vi "2024_day05.vi"() -> ()   [LabVIEW 2023]
uses:
  <userlib>/_OpenG.lib/array/array.llb/Search 1D Array (I32)__ogtk.vi
  <userlib>/_OpenG.lib/string/string.llb/openg_string.lvlib
  <userlib>/_OpenG.lib/array/array.llb/openg_array.lvlib
panel:
  out "Result - Task 2":i32
  out "Result - Task 1":i32
  in  "Switch":bool caption="Ex. Data  vs.  User Data"
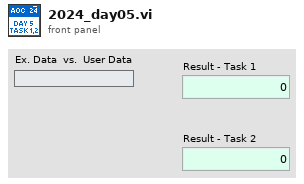
[diagram p1: front panel]
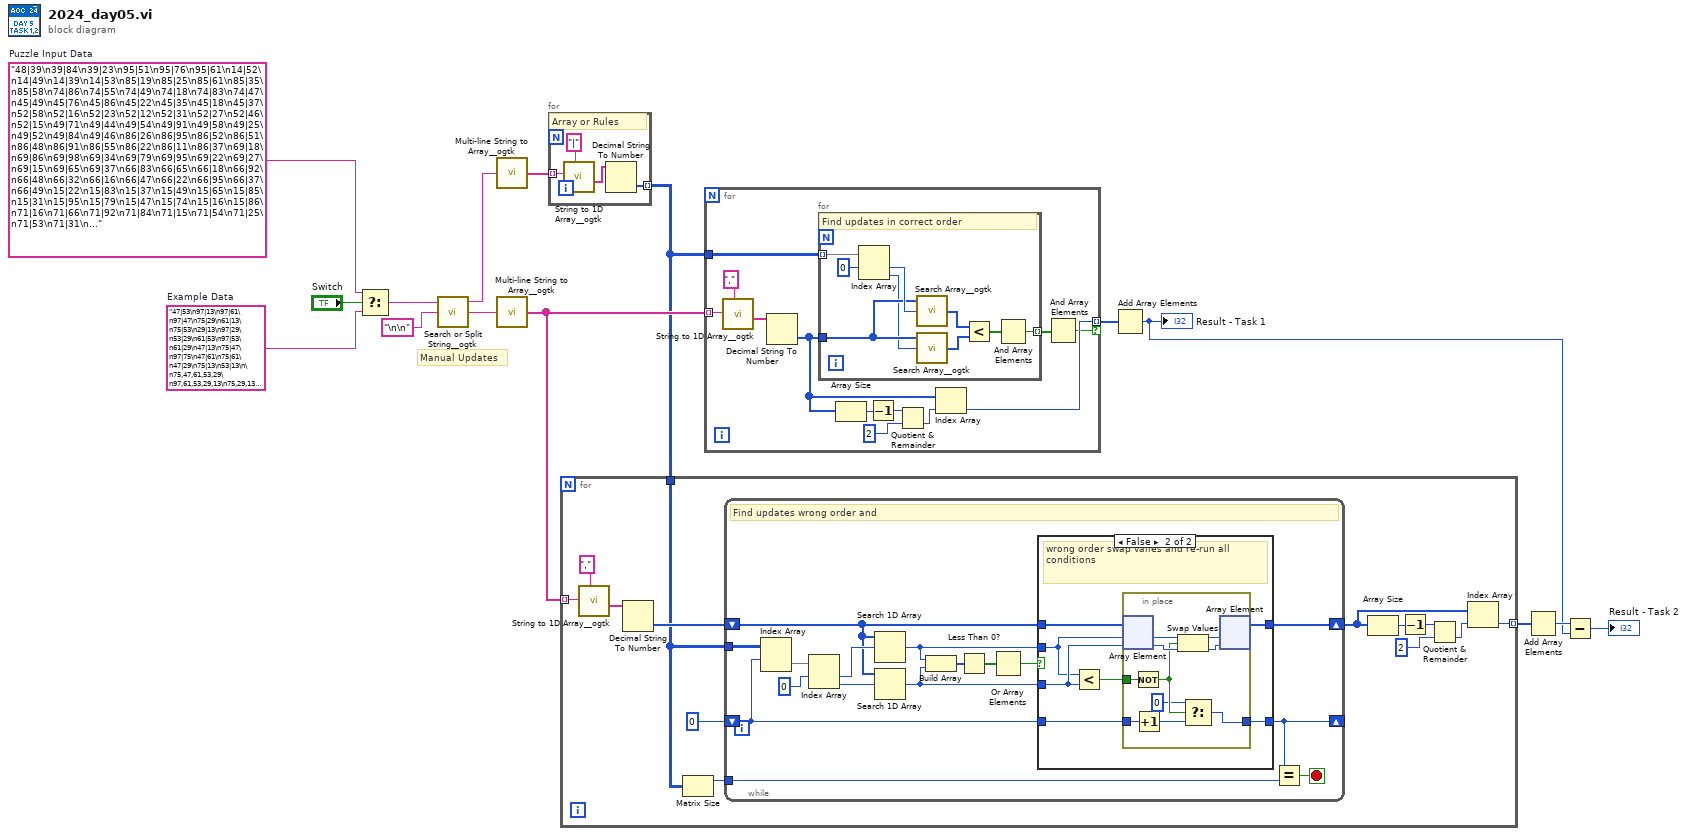
[diagram p0: block diagram]
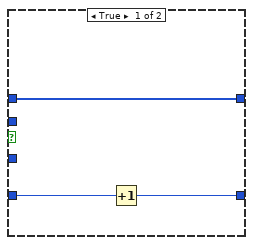
[diagram p2: hidden frame]
diagram:
  w13 = "48|39\n39|84\n39|23\n95|51\n95|76\n95|61\n14|52\n14|49\n14|39\n14|53\n85|19\n85|25\n85|61\n85|35\n85|58\n74|86\n74|55\n74|49\n74|18\n74|83\n74|47\n45|49\n45|76\n45|86\n45|22\n45|35\n45|18\n45|37\n52|58\n52|16\n52|23\n52|12\n52|31\n52|27\n52|46\n52|15\n49|71\n49|44\n49|54\n49|91\n49|58\n49|25\n49|52\n49|84\n49|46\n86|26\n86|95\n86|52\n86|51\n86|48\n86|91\n86|55\n86|22\n86|11\n86|37\n69|18\n69|86\n69|98\n69|34\n69|79\n69|95\n69|22\n69|27\n69|15\n69|65\n69|37\n66|83\n66|65\n66|18\n66|92\n66|48\n66|32\n66|16\n66|47\n66|22\n66|95\n66|37\n66|49\n15|22\n15|83\n15|37\n15|49\n15|65\n15|85\n15|31\n15|95\n15|79\n15|47\n15|74\n15|16\n15|86\n71|16\n71|66\n71|92\n71|84\n71|15\n71|54\n71|25\n71|53\n71|31\n71|98\n71|46\n71|69\n71|74\n71|58\n79|49\n79|34\n79|86\n79|26\n79|18\n79|14\n79|22\n79|91\n79|77\n79|48\n79|37\n79|52\n79|95\n79|35\n79|74\n76|39\n76|84\n76|94\n76|77\n76|12\n76|24\n76|46\n76|69\n76|15\n76|53\n76|23\n76|19\n76|52\n76|11\n76|66\n76|25\n19|94\n19|79\n19|71\n19|92\n19|66\n19|16\n19|53\n19|45\n19|69\n19|31\n19|24\n19|25\n19|12\n19|54\n19|84\n19|58\n19|98\n11|25\n11|27\n11|84\n11|12\n11|24\n11|66\n11|19\n11|51\n11|69\n11|16\n11|53\n11|94\n11|58\n11|44\n11|23\n11|39\n11|35\n11|52\n92|37\n92|91\n92|31\n92|48\n92|76\n92|14\n92|34\n92|55\n92|32\n92|85\n92|86\n92|98\n92|83\n92|49\n92|18\n92|26\n92|95\n92|11\n92|74\n23|16\n23|18\n23|86\n23|74\n23|92\n23|66\n23|79\n23|55\n23|45\n23|47\n23|26\n23|37\n23|15\n23|24\n23|12\n23|98\n23|34\n23|48\n23|65\n23|27\n37|51\n37|61\n37|26\n37|47\n37|49\n37|84\n37|52\n37|34\n37|55\n37|39\n37|14\n37|19\n37|77\n37|35\n37|58\n37|91\n37|83\n37|76\n37|85\n37|11\n37|32\n55|44\n55|19\n55|52\n55|39\n55|84\n55|54\n55|32\n55|47\n55|71\n55|51\n55|83\n55|35\n55|91\n55|85\n55|76\n55|11\n55|58\n55|61\n55|53\n55|49\n55|25\n55|77\n27|48\n27|18\n27|65\n27|34\n27|74\n27|37\n27|47\n27|98\n27|55\n27|83\n27|79\n27|16\n27|86\n27|85\n27|45\n27|66\n27|22\n27|49\n27|15\n27|26\n27|14\n27|92\n27|95\n51|16\n51|84\n51|54\n51|77\n51|27\n51|94\n51|66\n51|23\n51|19\n51|25\n51|71\n51|65\n51|15\n51|52\n51|39\n51|44\n51|46\n51|24\n51|12\n51|31\n51|92\n51|69\n51|58\n51|53\n83|32\n83|52\n83|35\n83|76\n83|94\n83|44\n83|84\n83|14\n83|71\n83|77\n83|61\n83|12\n83|85\n83|23\n83|39\n83|51\n83|19\n83|54\n83|25\n83|49\n83|11\n83|53\n83|58\n83|91\n94|66\n94|15\n94|74\n94|12\n94|55\n94|86\n94|16\n94|69\n94|26\n94|45\n94|34\n94|65\n94|98\n94|18\n94|23\n94|48\n94|46\n94|92\n94|37\n94|31\n94|22\n94|27\n94|24\n94|79\n54|15\n54|26\n54|92\n54|46\n54|69\n54|22\n54|23\n54|66\n54|24\n54|74\n54|31\n54|37\n54|16\n54|48\n54|34\n54|94\n54|65\n54|79\n54|45\n54|18\n54|12\n54|27\n54|86\n54|98\n58|23\n58|31\n58|48\n58|25\n58|79\n58|65\n58|15\n58|24\n58|16\n58|54\n58|86\n58|22\n58|94\n58|46\n58|27\n58|12\n58|45\n58|69\n58|92\n58|74\n58|66\n58|44\n58|98\n58|18\n61|65\n61|46\n61|54\n61|19\n61|77\n61|52\n61|39\n61|25\n61|66\n61|12\n61|24\n61|94\n61|44\n61|51\n61|27\n61|15\n61|69\n61|71\n61|23\n61|84\n61|58\n61|92\n61|16\n61|53\n77|53\n77|84\n77|24\n77|58\n77|65\n77|12\n77|31\n77|92\n77|46\n77|23\n77|66\n77|27\n77|25\n77|39\n77|19\n77|71\n77|16\n77|45\n77|52\n77|94\n77|69\n77|44\n77|54\n77|15\n32|35\n32|61\n32|51\n32|71\n32|91\n32|53\n32|46\n32|39\n32|52\n32|11\n32|23\n32|77\n32|76\n32|12\n32|27\n32|54\n32|94\n32|19\n32|58\n32|44\n32|25\n32|24\n32|69\n32|84\n31|85\n31|79\n31|35\n31|91\n31|86\n31|18\n31|76\n31|98\n31|55\n31|45\n31|95\n31|11\n31|49\n31|22\n31|14\n31|74\n31|34\n31|32\n31|26\n31|48\n31|83\n31|61\n31|37\n31|47\n34|26\n34|77\n34|85\n34|47\n34|61\n34|52\n34|19\n34|11\n34|58\n34|91\n34|35\n34|95\n34|39\n34|25\n34|14\n34|53\n34|71\n34|84\n34|76\n34|51\n34|83\n34|55\n34|49\n34|32\n46|22\n46|26\n46|98\n46|27\n46|45\n46|15\n46|83\n46|86\n46|24\n46|18\n46|65\n46|79\n46|34\n46|16\n46|55\n46|74\n46|95\n46|66\n46|92\n46|37\n46|47\n46|48\n46|69\n46|31\n26|53\n26|95\n26|35\n26|47\n26|19\n26|76\n26|83\n26|55\n26|11\n26|51\n26|77\n26|52\n26|39\n26|71\n26|91\n26|44\n26|32\n26|84\n26|85\n26|14\n26|49\n26|61\n26|25\n26|58\n91|24\n91|23\n91|94\n91|69\n91|46\n91|27\n91|76\n91|58\n91|53\n91|11\n91|19\n91|39\n91|52\n91|61\n91|84\n91|51\n91|25\n91|54\n91|77\n91|35\n91|44\n91|12\n91|15\n91|71\n53|48\n53|69\n53|44\n53|94\n53|92\n53|66\n53|79\n53|98\n53|31\n53|27\n53|45\n53|15\n53|16\n53|22\n53|12\n53|86\n53|54\n53|24\n53|58\n53|23\n53|74\n53|46\n53|65\n53|25\n12|74\n12|16\n12|65\n12|66\n12|95\n12|31\n12|34\n12|37\n12|47\n12|24\n12|98\n12|92\n12|15\n12|22\n12|69\n12|86\n12|27\n12|46\n12|55\n12|26\n12|45\n12|18\n12|79\n12|48\n24|34\n24|15\n24|26\n24|27\n24|95\n24|55\n24|37\n24|14\n24|74\n24|48\n24|31\n24|66\n24|45\n24|98\n24|18\n24|86\n24|92\n24|16\n24|65\n24|47\n24|83\n24|79\n24|22\n24|85\n84|54\n84|98\n84|53\n84|46\n84|58\n84|23\n84|22\n84|12\n84|16\n84|94\n84|45\n84|66\n84|65\n84|31\n84|86\n84|79\n84|25\n84|24\n84|69\n84|15\n84|74\n84|27\n84|92\n84|44\n18|53\n18|35\n18|55\n18|77\n18|85\n18|37\n18|83\n18|26\n18|52\n18|14\n18|39\n18|51\n18|19\n18|71\n18|11\n18|84\n18|91\n18|49\n18|32\n18|34\n18|76\n18|95\n18|61\n18|47\n25|65\n25|12\n25|94\n25|37\n25|45\n25|24\n25|92\n25|66\n25|79\n25|74\n25|22\n25|86\n25|98\n25|18\n25|44\n25|48\n25|23\n25|27\n25|16\n25|69\n25|31\n25|46\n25|54\n25|15\n98|83\n98|11\n98|22\n98|49\n98|37\n98|61\n98|85\n98|79\n98|95\n98|32\n98|35\n98|34\n98|48\n98|76\n98|77\n98|91\n98|47\n98|74\n98|86\n98|26\n98|51\n98|14\n98|18\n98|55\n22|76\n22|61\n22|47\n22|35\n22|85\n22|77\n22|51\n22|95\n22|26\n22|14\n22|37\n22|71\n22|83\n22|32\n22|55\n22|39\n22|52\n22|49\n22|91\n22|19\n22|18\n22|34\n22|11\n22|48\n47|95\n47|11\n47|14\n47|51\n47|49\n47|54\n47|39\n47|94\n47|85\n47|44\n47|61\n47|71\n47|58\n47|83\n47|19\n47|32\n47|77\n47|25\n47|84\n47|53\n47|76\n47|52\n47|35\n47|91\n35|54\n35|27\n35|77\n35|84\n35|71\n35|46\n35|12\n35|16\n35|51\n35|39\n35|52\n35|61\n35|15\n35|92\n35|94\n35|53\n35|66\n35|58\n35|44\n35|19\n35|25\n35|24\n35|23\n35|69\n65|45\n65|86\n65|95\n65|83\n65|31\n65|11\n65|35\n65|34\n65|18\n65|74\n65|32\n65|91\n65|26\n65|22\n65|49\n65|37\n65|14\n65|79\n65|55\n65|85\n65|76\n65|47\n65|98\n65|48\n44|74\n44|16\n44|86\n44|27\n44|48\n44|24\n44|94\n44|15\n44|65\n44|69\n44|66\n44|12\n44|22\n44|34\n44|23\n44|79\n44|92\n44|98\n44|31\n44|37\n44|18\n44|54\n44|45\n44|46\n16|18\n16|55\n16|92\n16|22\n16|79\n16|98\n16|26\n16|74\n16|45\n16|86\n16|76\n16|31\n16|47\n16|32\n16|83\n16|91\n16|48\n16|49\n16|85\n16|34\n16|65\n16|14\n16|95\n16|37\n48|71\n48|61\n48|52\n48|95\n48|76\n48|37\n48|91\n48|51\n48|77\n48|84\n48|34\n48|49\n48|18\n48|83\n48|11\n48|47\n48|26\n48|35\n48|32\n48|55\n48|14\n48|85\n48|19\n39|15\n39|65\n39|79\n39|19\n39|69\n39|53\n39|44\n39|31\n39|45\n39|54\n39|46\n39|92\n39|98\n39|16\n39|24\n39|58\n39|94\n39|25\n39|71\n39|66\n39|12\n39|27\n95|58\n95|11\n95|39\n95|44\n95|19\n95|94\n95|35\n95|83\n95|71\n95|91\n95|54\n95|77\n95|53\n95|52\n95|14\n95|84\n95|49\n95|85\n95|32\n95|23\n95|25\n14|35\n14|76\n14|94\n14|25\n14|46\n14|58\n14|84\n14|23\n14|11\n14|71\n14|12\n14|77\n14|32\n14|19\n14|61\n14|44\n14|54\n14|85\n14|91\n14|51\n85|53\n85|49\n85|76\n85|71\n85|44\n85|94\n85|11\n85|12\n85|39\n85|91\n85|77\n85|52\n85|54\n85|69\n85|46\n85|23\n85|51\n85|84\n85|32\n74|61\n74|95\n74|26\n74|91\n74|48\n74|14\n74|37\n74|52\n74|34\n74|39\n74|32\n74|77\n74|22\n74|51\n74|76\n74|35\n74|11\n74|85\n45|83\n45|91\n45|11\n45|51\n45|79\n45|34\n45|47\n45|98\n45|55\n45|14\n45|74\n45|48\n45|26\n45|61\n45|32\n45|85\n45|95\n52|19\n52|98\n52|54\n52|71\n52|45\n52|25\n52|65\n52|92\n52|53\n52|66\n52|39\n52|84\n52|94\n52|69\n52|24\n52|44\n49|23\n49|11\n49|39\n49|51\n49|53\n49|35\n49|61\n49|24\n49|19\n49|94\n49|12\n49|77\n49|32\n49|69\n49|76\n86|49\n86|14\n86|83\n86|32\n86|76\n86|85\n86|61\n86|77\n86|18\n86|19\n86|34\n86|35\n86|47\n86|39\n69|92\n69|16\n69|83\n69|66\n69|48\n69|24\n69|26\n69|47\n69|14\n69|45\n69|55\n69|74\n69|31\n66|26\n66|79\n66|91\n66|31\n66|34\n66|85\n66|45\n66|98\n66|86\n66|14\n66|55\n66|74\n15|45\n15|14\n15|26\n15|32\n15|18\n15|98\n15|48\n15|34\n15|66\n15|92\n15|55\n71|45\n71|24\n71|44\n71|86\n71|12\n71|79\n71|23\n71|65\n71|94\n71|27\n79|85\n79|55\n79|11\n79|83\n79|61\n79|51\n79|76\n79|47\n79|32\n76|51\n76|27\n76|44\n76|35\n76|54\n76|58\n76|61\n76|71\n19|65\n19|23\n19|46\n19|15\n19|27\n19|74\n19|44\n11|61\n11|15\n11|77\n11|71\n11|54\n11|46\n92|47\n92|22\n92|79\n92|45\n92|65\n23|46\n23|22\n23|69\n23|31\n37|95\n37|53\n37|71\n55|95\n55|14\n27|31\n\n61,58,51,32,12,14,71\n58,25,54,14,12,94,32,76,39\n35,53,26,77,14,71,25,76,85,55,51,49,95\n32,91,76,11,35,61,51,77,52,19,71,84,53,58,25,44,54,94,23,12,46,69,24\n18,37,26,47,83,85,49,32,76,35,61,77,52,19,71\n39,19,84,53,58,25,54,12,69,66,31\n61,52,71,84,44,66,92\n71,84,44,46,45\n32,91,76,35,51,77,52,71,84,53,58,25,44,54,94,23,12\n48,18,37,34,26,55,47,95,83,49,32,91,11,35,61,77,52,39,71\n25,54,12,46,79,74,18\n94,65,44,39,46,66,52,15,54,71,84,92,12,77,23,27,31,16,25,58,19,69,53\n19,71,53,25,44,54,94,23,46,69,24,15,66,16,65,31,79\n49,76,11,35,77,52,39,71,54,23,12,46,69\n69,58,19,71,35,61,16,46,54\n54,16,35,94,25,15,51\n34,26,55,47,95,14,85,49,32,91,76,11,35,61,51,77,52,39,19,71,84,53,58\n76,54,77,24,46,12,27,35,53,52,61,39,58,69,94,71,91,23,51\n14,27,83,85,37,65,16,18,79,22,48,66,86,92,47\n19,52,61,58,44,84,51\n27,15,66,16,92,31,98,79,74,86,18,37,26,55,85\n94,46,27,66,65,45,98,74,86,48,18,37,34\n66,46,53,52,77,35,16,27,61\n18,37,34,55,47,95,83,14,85,49,32,91,76,11,35,61,51,77,39,71,84\n61,51,77,52,39,19,71,84,53,58,25,54,94,23,12,46,69,24,27,15,66,16,92\n98,74,86,22,48,18,37,34,26,55,47,95,83,14,85,49,32,91,76,11,51\n49,32,51,39,84,53,69\n46,15,66,65,45,98,86,48,18,34,55,47,95\n25,94,23,12,66,16,92,31,79,86,22,48,18\n32,91,76,51,77,52,39,19,53,58,25,54,94,23,12,69,24\n34,26,55,47,83,14,76,35,61,51,77,39,19,84,53\n34,18,95,74,35,37,47,52,76,32,22,48,51,86,77,85,11,55,83,14,26\n25,44,54,23,46,69,27,16,92,31,45,98,22,48,18\n91,58,11,76,26,49,19,95,14,61,39\n48,18,37,34,55,47,95,14,85,49,32,91,76,35,61,51,77,52,39,19,71\n31,66,27,79,23,86,22,92,15,44,54,94,16,37,12,18,45\n16,24,66,53,12,77,19,65,15,51,27,94,23,52,39,46,58,69,92,84,71,54,25\n44,54,94,12,46,24,27,15,92,31,86,22,37\n39,71,53,54,15,45,98\n69,53,44,54,77,58,27,39,61,25,12,94,23,51,35,84,71,15,46,66,16,19,52\n94,46,69,31,66,84,86,58,98,16,24\n55,47,95,49,76,51,19,71,84,58,44\n12,46,69,16,92,65,31,45,98,79,74,86,22,48,18,37,34,26,47\n52,11,77,58,27,35,39,24,44,19,46,23,54,53,71,76,12\n71,66,94,15,84,46,61,52,11,19,53,23,51,69,27,54,58,12,39,44,24\n79,86,22,18,37,47,83,14,91,76,51\n79,48,47,95,11\n12,24,46,34,66,74,86,98,69,37,45,92,26,55,47,18,65,22,16\n71,65,54,15,39,69,98,23,46,58,94,24,45\n79,74,86,83,14\n35,19,84,69,27\n54,46,66,31,98,48,18,37,34\n18,65,34,14,55,66,24\n94,46,27,65,98,22,26\n66,69,45,46,79,23,86,92,58,94,84,53,24,31,44,54,16,12,65,27,98\n27,66,92,65,31,98,86,18,26,55,95,83,85\n86,34,79,83,66,55,22,16,32\n85,49,32,76,11,77,52,39,84,53,25,54,94,12,46\n74,47,31,22,92,18,79,37,48,14,16,85,98,83,34,45,65,95,66,27,86\n86,22,18,37,34,26,47,95,83,85,49,32,11,35,61,77,39\n79,55,95,49,91\n54,94,23,12,46,69,24,27,15,66,16,65,31,45,98,79,74,86,22,48,18,37,34\n27,53,58,92,69,79,94\n83,14,85,49,32,91,76,11,35,61,51,77,52,39,19,71,84,53,58,44,54,94,23\n23,12,46,69,24,27,15,66,16,92,65,31,98,79,74,86,22,48,18,37,34,26,55\n53,54,19,85,46,91,84,71,44,52,23,51,77,76,39,32,25,94,49,11,61\n32,35,55,22,74\n35,61,51,77,39,19,71,84,53,58,25,44,54,94,23,12,46,69,24,27,15,66,16\n95,74,11,49,85,83,45,34,32,61,37,35,14,55,18,79,26,22,98,86,91,47,48\n66,31,45,98,22,48,47,95,83,14,85\n61,51,77,52,39,19,71,84,53,58,25,54,94,23,12,46,69,27,15,16,92\n85,49,91,35,61,77,52,39,19,71,84,53,58,25,94,12,46\n47,26,79,65,34,37,74,83,98,22,45,55,18,16,66,69,15,86,95\n61,51,46,23,12,25,85,58,52,39,54,19,76,91,94,32,35\n48,37,95,85,32,91,76,51,71\n84,58,25,44,54,94,23,12,46,69,24,27,15,66,16,92,65,31,98,79,86\n77,54,14,35,49,84,76,51,11,44,94,95,52,71,19\n69,24,27,15,66,16,92,65,31,45,98,79,74,22,48,18,37,34,26,55,47,95,83\n61,71,53,44,46,24,66\n66,16,45,18,55,47,83,85,32\n69,24,27,66,98,79,86,22,48,18,37,34,26,55,47,95,83\n85,19,71,84,44,11,53,47,77,49,76,54,14,91,25\n11,83,61,77,51,35,58,94,95\n49,32,91,76,11,35,61,51,77,52,39,19,84,58,25,44,94,23,12,46,69\n25,44,54,94,23,12,24,27,15,66,16,92,65,31,79,74,86,22,18\n71,49,48,95,76,83,34,47,37\n14,49,32,91,61,77,52,19,84,58,44\n45,44,79,53,16,23,15,58,92,31,66,22,98,74,25,24,46,69,65,86,54,27,94\n11,61,52,53,58,94,66\n77,84,54,69,71,76,24,23,94,11,44,27,91,12,61,53,35,19,39,46,25\n92,65,31,45,74,86,48,18,37,34,26,55,47,95,83,14,85,91,76\n46,24,15,66,16,92,98,79,86,18,34,26,55\n11,35,61,51,77,52,39,19,71,53,58,25,44,54,94,23,12,69,24,15,66\n49,76,39,53,58\n71,84,53,58,25,44,54,94,23,12,69,24,27,15,66,16,92,65,31,45,98,79,74\n14,25,47,32,54,19,85,95,58\n53,12,25,19,15,54,52,31,44,39,69\n32,91,76,35,61,51,77,52,39,19,84,58,25,44,54,94,23,12,46,69,24\n55,83,91,49,86,22,76,37,32,14,39,47,34\n94,23,12,46,69,24,27,66,16,92,65,31,45,98,79,74,86,22,48,18,37,34,26\n55,83,49,32,35,39,19\n19,16,92,46,31,69,44,52,39,12,71,45,53,15,84,66,58\n71,84,35,53,58,11,91,61,51,83,25,14,47,77,32,76,44,55,95,52,19,49,39\n24,27,65,31,45,98,22,48,18,34,26,55,47,95,14\n46,23,58,31,98,12,92,24,45,54,71,94,19,16,53,25,39,44,69\n92,65,98,18,47,83,14,85,76\n26,32,34,83,49,91,52,85,47,11,51,76,74,35,48\n65,45,98,79,74,22,48,18,55,47,95,83,14,85,49,32,91,76,11\n47,39,26,22,49,34,76\n77,52,84,54,23,46,27,16,31\n15,66,16,92,65,31,98,74,86,48,18,37,34,55,47\n92,55,48,18,27,45,65,24,66,83,69\n22,18,37,95,85,49,32,35,61,77,19\n49,91,77,71,58,25,54,94,69\n39,51,85,77,49,19,61,18,22,37,14,34,11\n47,85,32,91,76,52,39,19,71,84,53,44,54\n76,35,61,52,39,71,53,58,25,94,12,46,24,27,15\n61,51,84,25,46,35,76,32,52,12,23,69,19,94,58,11,39,53,24,54,77,44,91\n31,45,66,49,79,95,26,98,65,48,14,55,22,74,92\n92,46,48,26,66\n25,44,94,12,65,31,79,22,18\n45,98,79,55,14,34,26,83,74,15,86,92,85,49,18,66,65,16,22\n25,32,53,58,94,23,19,54,71,11,39,77,52,84,69,76,49\n52,39,84,53,25,44,12,24,15,66,16,92,65,31,45\n52,39,19,58,44,54,94,23,12,69,24,15,66,16,92,31,45\n95,66,47,26,18,83,32,45,85,98,86,37,55\n31,45,86,48,37,26,95,83,14,85,32,76,35\n94,24,92,58,19,54,69,16,84,53,27,51,77,12,15,61,39,25,52,23,71,66,44\n44,54,94,23,12,46,69,24,66,92,31,98,79\n66,16,92,65,45,98,79,74,86,22,48,18,37,26,55,47,95,83,14,49,32\n98,18,47,14,85,49,51\n55,85,91,11,84\n32,91,11,35,51,77,52,39,19,84,58,54,94,23,69\n83,84,11,26,77,34,14,85,71,52,18\n32,49,91,76,83,94,71,19,23,61,58\n44,69,16,98,65,58,12,84,94,25,79,27,31,54,46,24,86,66,74,45,92\n65,94,15,12,45,74,23,58,16,84,86,31,69,24,98,92,66\n61,51,77,52,19,71,84,53,25,44,94,23,12,46,69,24,27,15,66\n79,34,55,61,98,45,47,74,83,49,76,11,32\n86,22,48,18,37,83,85,32,91,76,11,35,61,51,77,52,39\n65,45,86,55,95,85,32,76,11\n15,66,16,92,31,45,98,79,74,86,22,48,18,37,34,26,95,83,14,85,49\n54,58,53,16,71,15,98,69,94,65,46,31,66,25,92,84,44,24,19,23,27\n26,61,37,14,71,51,19,76,91\n15,92,79,74,86,22,48,26,55,83,14,85,49\n26,74,83,76,49,31,47,35,37,95,86\n71,83,95,34,19,39,14,51,85,49,52,61,32,48,55\n69,15,66,92,79,74,37,34,55,47,95\n47,51,19,39,35,85,84,91,26,71,49,55,25,11,52\n26,14,76,32,37,95,86,35,55,79,83,11,91,47,34,22,31,98,85,45,48\n35,53,19,32,91,46,12,25,11,61,54,51,71\n98,79,74,86,22,18,37,34,26,55,47,95,83,85,49,32,91,11,51\n79,22,34,47,32,11,77\n31,69,45,95,83,16,55,65,98,22,26,37,74\n74,86,22,37,34,26,55,95,85,32,91,76,11,77,52\n39,19,71,53,25,44,54,46,69,24,27,66,16,65,31,45,98\n47,51,11,77,58,85,52\n45,48,37,83,49,32,91\n85,26,77,95,19,18,51,34,55,52,91,32,11,84,39\n79,45,18,94,48,74,16,12,92,98,37,26,27,23,69,46,34,86,31\n48,34,14,45,86,98,18,85,47,22,55,76,79,32,31,91,35,83,37\n76,77,52,71,44\n26,55,47,95,83,14,85,49,32,91,76,11,35,61,51,77,52,39,19,71,84,58,25\n45,98,79,86,48,18,34,26,47,95,85,91,61\n24,44,19,71,15,12,27,51,52,92,84\n69,24,27,65,98,22,48,18,55,47,83\n61,34,11,74,91,51,48,55,52,86,37,85,14,49,95,76,22\n71,46,27,15,66,92,79\n58,46,16,31,27,54,53,66,12,23,71,52,84,25,44,94,77\n61,77,39,19,71,84,25,44,54,94,24,27,15,66,16\n51,52,15,12,24,66,54,35,46,16,69,84,53\n74,86,22,48,18,34,26,55,47,95,83,14,85,49,32,91,76,11,35,61,51,77,52\n34,26,47,14,32,76,35,39,71\n37,26,47,83,85,49,76,11,35,61,51,77,53\n66,24,98,86,15\n91,76,35,61,51,52,39,19,53,58,54,94,23,46,27\n16,92,45,74,86,22,18,37,34,26,55,85,49,32,91\n12,74,58,79,23,31,22,25,86\n98,79,22,48,18,14,85,49,32,76,11,61,51\n34,26,55,47,95,83,14,85,49,32,91,76,11,35,61,51,52,39,19,71,84,53,58\n51,52,39,58,25,44,54,12,46,69,24,66,16,92,65\n24,44,58,12,46,92,22,79,86,74,54,65,23\n86,22,18,26,95,32,91,76,51\n71,54,69,24,15,66,16,31,45,98,74\n15,92,65,31,45,98,79,74,86,22,48,18,34,26,55,95,14,85,49\n53,44,54,94,23,12,46,69,24,27,15,66,92,98,74,86,22\n16,92,65,31,45,98,22,18,37,34,55,95,83,14,32\n34,47,95,83,14,85,49,91,76,11,35,51,77,52,19,71,84,53,58\n55,45,76,37,35,83,31"  # Puzzle Input Data
  w14 = "47|53\n97|13\n97|61\n97|47\n75|29\n61|13\n75|53\n29|13\n97|29\n53|29\n61|53\n97|53\n61|29\n47|13\n75|47\n97|75\n47|61\n75|61\n47|29\n75|13\n53|13\n\n75,47,61,53,29\n97,61,53,29,13\n75,29,13\n75,97,47,61,53\n61,13,29\n97,13,75,29,47"  # Example Data
  # "Manual Updates"
  n1 = Select(t=w13, s="Switch", f=w14) -> (s? t:f=w12:string)
  n2 = call <userlib>:"Search or Split String__ogtk.vi"("search string/char (-)"="\n\n", "string"=w12) -> ("substring after match"=w10:string, "substring before match"=w9:string)  [unwired: 1 in, 1 out]
  n3 = call <userlib>:"Multi-line String to Array__ogtk.vi"("string"=w9) -> ("lines"=w8:string[])
  n4 = call <userlib>:"Multi-line String to Array__ogtk.vi"("string"=w10) -> ("lines"=w5:string[])
  n5 = for {
    tunnel: w8 -> [w18] mode=indexing
    tunnel: [w16] -> w4 mode=indexing
    # "Array or Rules"
    n6 = call <userlib>:"String to 1D Array__ogtk.vi"("delimiter (Tab)"="|", "string"=w18) -> ("Array of Strings"=w17:string[])  [unwired: 9 in]
    n7 = Decimal String To Number(string=w17) -> (number=w16:i32[])  [unwired: 2 in, 1 out]
  }
  n8 = for {
    tunnel: w5 -> [w32] mode=indexing
    tunnel: w4 -> [w20]
    tunnel: [w25] -> w6 mode=indexing
    n9 = call <userlib>:"String to 1D Array__ogtk.vi"("delimiter (Tab)"=",", "string"=w32) -> ("Array of Strings"=w30:string[])  [unwired: 9 in]
    n10 = Decimal String To Number(string=w30) -> (number=w22:i32[])  [unwired: 2 in, 1 out]
    n11 = Matrix Size(0:w20) -> (1:w21:i32)  [unwired: 1 out]
    n12 = while {
      tunnel: w20 -> [w43]
      shift-right: [w44] -> w23
      shift-left: w22 -> [w45]
      shift-right: [w39] -> _
      shift-left: 0 ("index") -> [w42]
      tunnel: w21 -> [w38]
      stop <- w40 stop-if-true
      # "Find updates wrong order and"
      n13 = Index Array(array=w43, index (row)=w42) -> (element=w41:i32[])  [unwired: 1 in]
      n14 = Index Array(array=w41, index #1=0 ("index")) -> (element #1=w48:i32, element #2=w46:i32)  [unwired: 1 in]
      n15 = Search 1D Array(1D array=w45, element=w48) -> (index of element=w37:i32)  [unwired: 1 in]
      n16 = Search 1D Array(1D array=w45, element=w46) -> (index of element=w36:i32)  [unwired: 1 in]
      n17 = Build Array(w37, w36) -> (w35:i32[])
      n18 = Less Than 0?(x=w35) -> (x < 0?=w34:bool[])
      n19 = Or Array Elements(Boolean array=w34) -> (logical OR=w33:bool)
      n20 = case shown="False" w33 {
        tunnel: w45 -> [w49 w58]
        tunnel: [w49 w57] -> w44
        tunnel: w42 -> [w51 w55]
        tunnel: w36 -> [_ w53]
        tunnel: [w50 w56] -> w39
        tunnel: w37 -> [_ w52]
        frame True {
          n21 = Increment(x=w51) -> (x+1=w50:i32)
        }
        frame False {
          # "wrong order swap valies and re-run all conditions"
          n22 = Less?(x=w52, y=w53) -> (x < y?=w54:bool)
          n23 = in-place {
            in-place-border: w54 -> [w64]
            in-place-border: w55 -> [w62]
            in-place-border: [w63] -> w56
            n24 = in-place-array #1(w58, w52, w53) -> (w68:i32, w67:i32)
            n25 = Not(x=w64) -> (.not. x?=w60:bool)
            n26 = Increment(x=w62) -> (x+1=w61:i32)
            n27 = Swap Values(12:w68, 13:w60, 14:w67) -> (1:w66:i32, 3:w65:i32)
            n28 = Select(t=0 ("index"), s=w60, f=w61) -> (s? t:f=w63:i32)
            n29 = in-place-array #1(w66, w65) -> (w57:i32[])  [unwired: 2 out]
          }
        }
      }
      n30 = Equal?(x=w39, y=w38) -> (x = y?=w40:bool)
    }
    n31 = Array Size(array=w23) -> (size(s)=w29:i32)
    n32 = Decrement(x=w29) -> (x-1=w27:i32)
    n33 = Quotient & Remainder(x=w27, y=2) -> (floor(x/y)=w26:i32)  [unwired: 1 out]
    n34 = Index Array(array=w23, index=w26) -> (element=w25:i32)
  }
  n35 = for {
    tunnel: w5 -> [w80] mode=indexing
    tunnel: w4 -> [w77]
    tunnel: [w70] -> w7 mode=indexing if=w69
    n36 = call <userlib>:"String to 1D Array__ogtk.vi"("delimiter (Tab)"=",", "string"=w80) -> ("Array of Strings"=w78:string[])  [unwired: 9 in]
    n37 = Decimal String To Number(string=w78) -> (number=w72:i32[])  [unwired: 2 in, 1 out]
    n38 = for {
      tunnel: w77 -> [w89] mode=indexing
      tunnel: w72 -> [w86]
      tunnel: [w81] -> w76 mode=indexing
      # "Find updates in correct order"
      n39 = Index Array(array=w89, index #1=0 ("index")) -> (element #1=w88:i32, element #2=w85:i32)  [unwired: 1 in]
      n40 = call-poly <userlib>:"Search Array__ogtk.vi"("Array"=w86, "Element Data"=w88) -> ("Indices of Elements"=w84:i32[])  [unwired: 7 in]
      n41 = call-poly <userlib>:"Search Array__ogtk.vi"("Array"=w86, "Element Data"=w85) -> ("Indices of Elements"=w83:i32[])  [unwired: 7 in]
      n42 = Less?(x=w84, y=w83) -> (x < y?=w82:bool[])
      n43 = And Array Elements(Boolean array=w82) -> (logical AND=w81:bool)
    }
    n44 = Array Size(array=w72) -> (size(s)=w75:i32)
    n45 = Decrement(x=w75) -> (x-1=w73:i32)
    n46 = Quotient & Remainder(x=w73, y=2) -> (floor(x/y)=w71:i32)  [unwired: 1 out]
    n47 = Index Array(array=w72, index=w71) -> (element=w70:i32)
    n48 = And Array Elements(Boolean array=w76) -> (logical AND=w69:bool)
  }
  n49 = Add Array Elements(numeric array=w7) -> (sum=w1:i32)
  "Result - Task 1" <- w1
  n50 = Add Array Elements(numeric array=w6) -> (sum=w3:i32)
  n51 = Subtract(x=w3, y=w1) -> (x-y=→"Result - Task 2":i32)
